vi "CMD_ReadBlueToothAddress.vi"(0 "Input_Data":string[](array[string]), 5 "Error In":errorcluster) -> (12 "Validate CheckSum":bool, 13 "Command":u8[](array[numeric])=[5, 247, 4, 128, 255, 0, 0, 0, 0, 0, 0, 0, 0, 0] format="%x", 14 "Response":bool, 15 "Ack":bool, 16 "Command":bool, 17 "Add CheckSum":bool, 18 "Status":bool, 19 "Error Out":errorcluster)   [LabVIEW 2014]
panel:
  # "Flags"
  # "Store BT Address Command:"
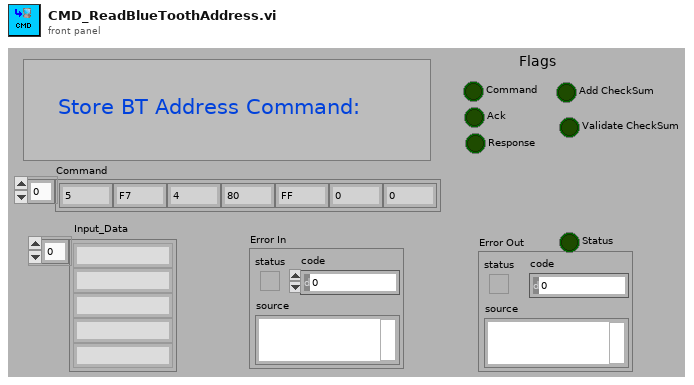
[diagram p1: front panel]
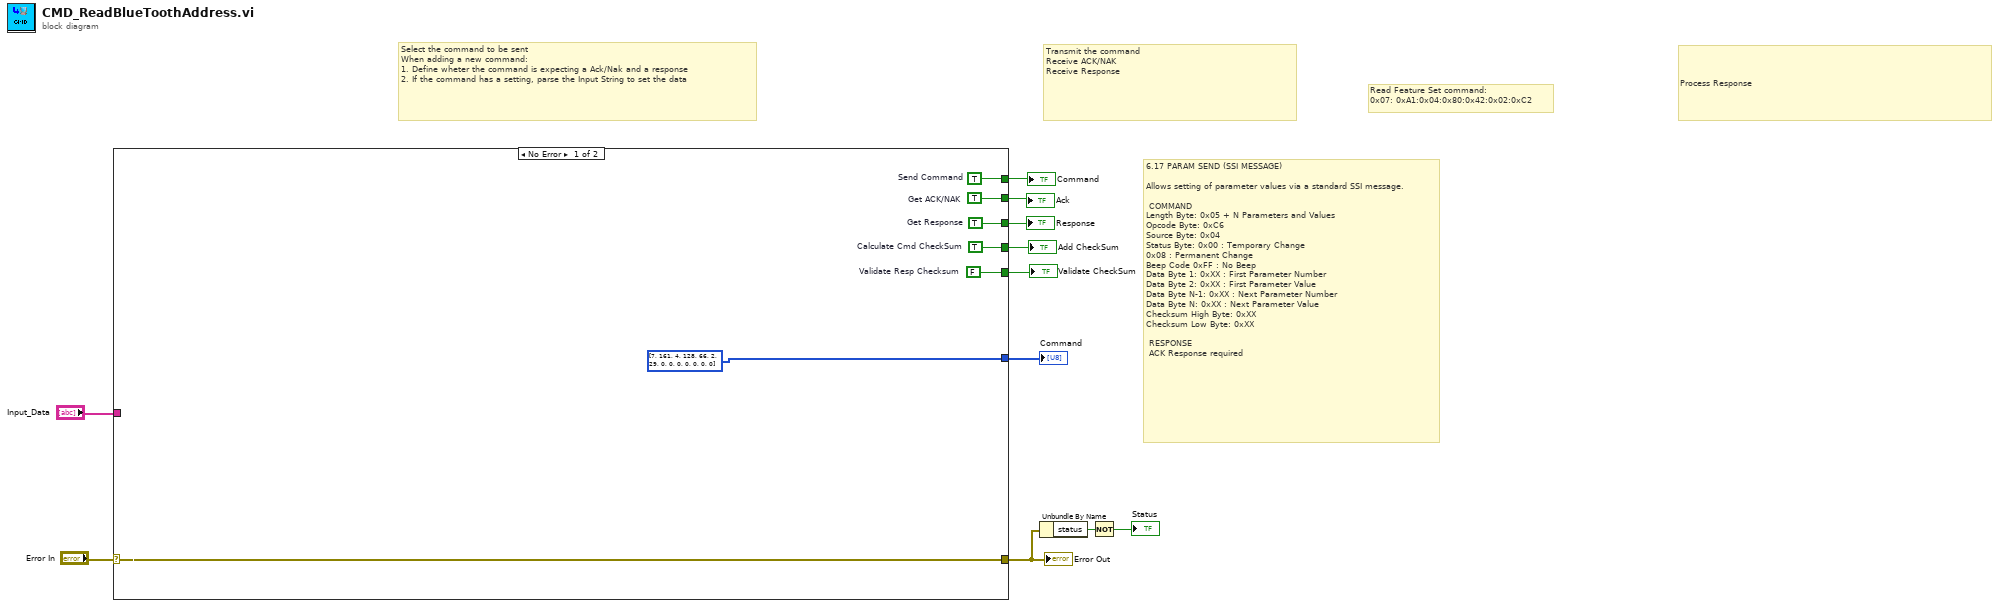
[diagram p0: block diagram]
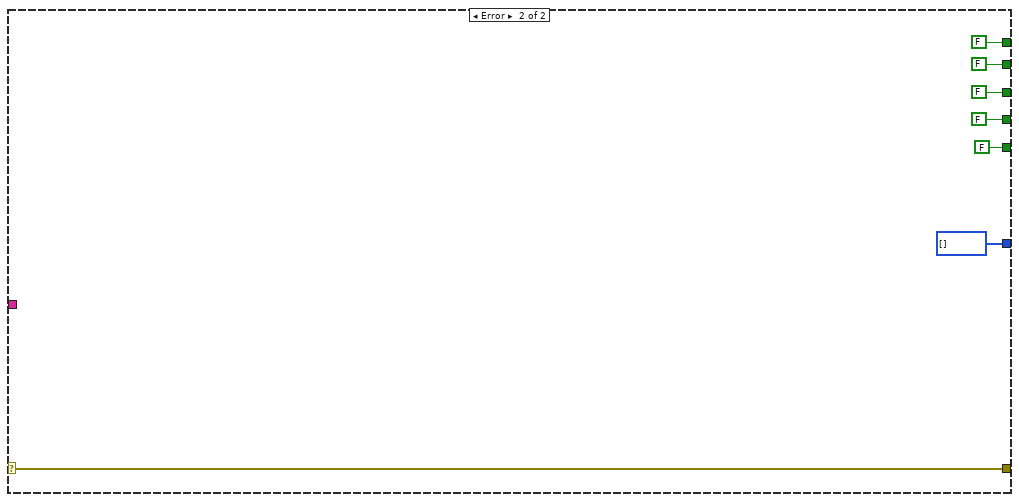
[diagram p2: hidden frame]
diagram:
  # "6.17\tPARAM SEND (SSI MESSAGE)\n\nAllows setting of parameter values via a standard SSI message.\n\n\tCOMMAND\nLength Byte:\t0x05 + N Parameters and Values\nOpcode Byte:\t0xC6\nSource Byte:\t0x04\nStatus Byte:\t0x00 : Temporary Change\n0x08 : Permanent Change\nBeep Code\t0xFF : No Beep\nData Byte 1:\t0xXX : First Parameter Number\nData Byte 2:\t0xXX : First Parameter Value\nData Byte N-1:\t0xXX : Next Parameter Number\nData Byte N:\t0xXX : Next Parameter Value\nChecksum High Byte:\t0xXX\nChecksum Low Byte:\t0xXX\n\n\tRESPONSE\n\tACK Response required"
  # "Read Feature Set command:\n0x07: 0xA1:0x04:0x80:0x42:0x02:0xC2"
  # "Process Response"
  # "Transmit the command\nReceive ACK/NAK\nReceive Response"
  # "Select the command to be sent\nWhen adding a new command:\n1. Define wheter the command is expecting a Ack/Nak and a response\n2. If the command has a setting, parse the Input String to set the data"
  n1 = case shown="No Error" "Error In" {
    selector: "Error In" -> [w14 w20]
    tunnel: [w18 FALSE ("Send Command")] -> w10
    tunnel: [w17 FALSE ("Get ACK/NAK")] -> w9
    tunnel: [w16 FALSE ("Get Response")] -> w8
    tunnel: [w15 FALSE ("Add CheckSum")] -> w7
    tunnel: [u8[] [7, 161, 4, 128, 66, 2, 29, 0, 0, 0, 0, 0, 0, 0] u8[] []] -> w1
    tunnel: [w14 w20] -> w5
    tunnel: "Input_Data" -> [_ _]
    tunnel: [w13 FALSE ("Validate Resp Checksum")] -> w2
    frame No Error {
      w13 = FALSE  # Validate Resp Checksum
      w15 = TRUE  # Calculate Cmd CheckSum
      w16 = TRUE  # Get Response
      w18 = TRUE  # Send Command
      w17 = TRUE  # Get ACK/NAK
    }
    frame Error {
    }
  }
  "Error Out" <- w5
  "Command" <- w10
  "Ack" <- w9
  "Response" <- w8
  "Add CheckSum" <- w7
  "Validate CheckSum" <- w2
  "Command" <- w1
  n2 = Unbundle By Name(w5) -> ("status"=w4:bool)
  n3 = Not(x=w4) -> (.not. x?=→"Status":bool)
